vi "GetDisplayBlinkingState.vi"(8 "Error In":errorcluster, 10 "Window":u8 min=1 max=2 step=1, 11 "Keithley 6482 In":refnum<visa-resource-name>) -> (0 "Error Out":errorcluster, 2 "Blinking?":bool, 3 "Keithley 6482 Out":refnum<visa-resource-name>)   [LabVIEW 2009, in "Keithley-6482-Visa.lvlib"]
uses:
  <instrlib>/Keithley-6482-Visa9.0/Keithley-6482-Visa.lvlib
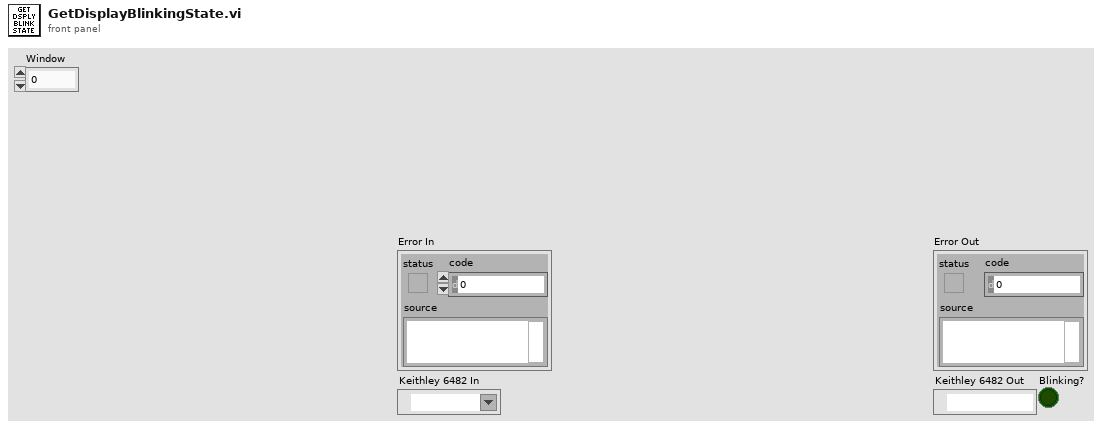
[diagram p1: front panel]
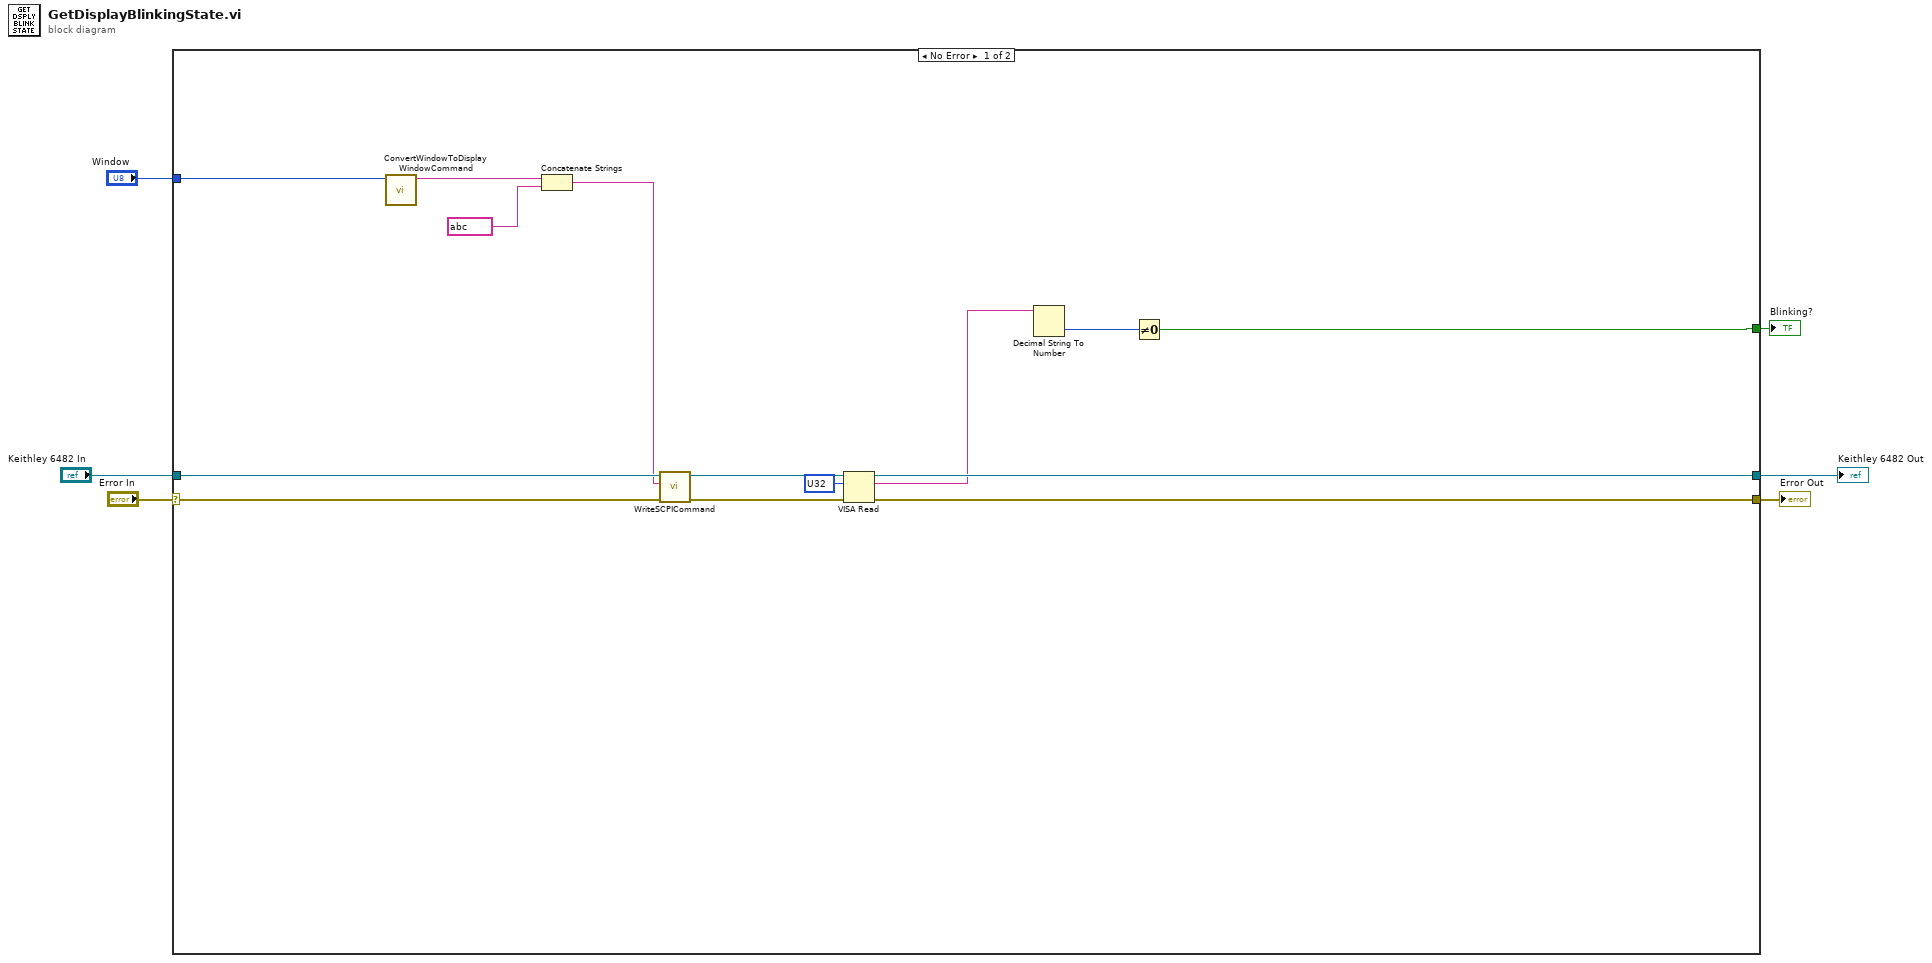
[diagram p0: block diagram]
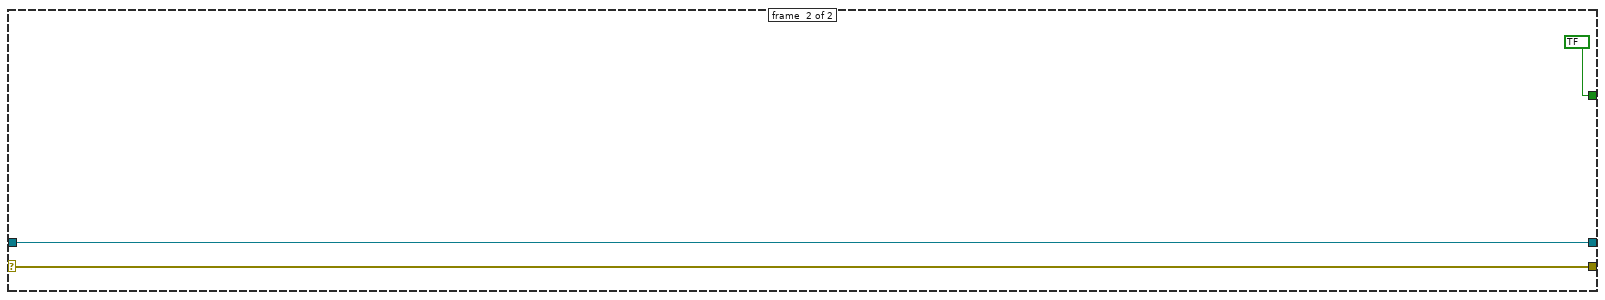
[diagram p2: hidden frame]
diagram:
  n1 = case shown="No Error" "Error In" {
    selector: "Error In" -> [w14 w22]
    tunnel: [w20 w22] -> w5
    tunnel: [w19 w23] -> w4
    tunnel: "Keithley 6482 In" -> [w15 w23]
    tunnel: [w11 bool ? ("Boolean")] -> w2
    tunnel: "Window" -> [w7 _]
    frame #0 {
      n2 = call <instrlib>:"ConvertWindowToDisplayWindowCommand.vi"("Window"=w7) -> ("Display Window Command"=w8:string)  [unwired: 10 in]
      n3 = Concatenate Strings(w8, string ?) -> (w9:string)
      n4 = call <instrlib>:"WriteSCPICommand.vi"("Error In"=w14, "SCPI Command"=w9, "Keithley 6482 In"=w15) -> ("Error Out"=w16:errorcluster, "Keithley 6482 Out"=w17:refnum<visa-resource-name>)  [unwired: 7 in]
      n5 = VISA Read(VISA resource name=w17, byte count=u32 ?, error in (no error)=w16) -> (VISA resource name out=w19:refnum<visa-resource-name>, read buffer=w13:string, error out=w20:errorcluster)  [unwired: 1 out]
      n6 = Decimal String To Number(string=w13) -> (number=w12:i32)  [unwired: 2 in, 1 out]
      n7 = Not Equal To 0?(x=w12) -> (x != 0?=w11:bool)
    }
    frame #1 {
    }
  }
  "Error Out" <- w5
  "Keithley 6482 Out" <- w4
  "Blinking?" <- w2
